vi "EncoderDistanceToDegrees.vi"(1 "Right Distance":dbl format="%#_13g", 2 "Left Distance":dbl format="%#_13g") -> (0 "Degrees":dbl)   [LabVIEW 2016]
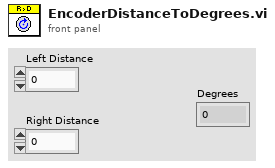
[diagram p1: front panel]
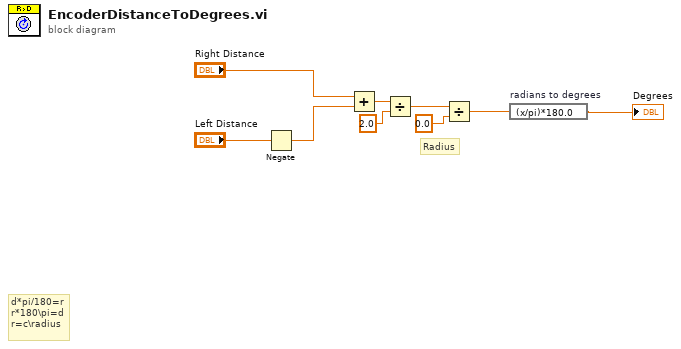
[diagram p0: block diagram]
diagram:
  # "d*pi/180=r\nr*180\\pi=d\nr=c\\radius"
  # "Radius"
  n1 = Negate(x="Left Distance") -> (-x=w7:dbl)
  n2 = Add(x="Right Distance", y=w7) -> (x+y=w6:dbl)
  n3 = Divide(x=w6, y=2.0) -> (x/y=w2:dbl)
  n4 = Divide(x=w2, y=0.0) -> (x/y=w3:dbl)
  n5 = expression code="(x/pi)*180.0" "radians to degrees"(w3) -> (→"Degrees":dbl)
